vi "Event_Shape_Identifier_2011.vi"() -> ()   [LabVIEW 2011]
uses:
  <vilib>/Analysis/NI_AALPro.lvlib
  <vilib>/Utility/file.llb/Read From Spreadsheet File (string).vi
  <vilib>/Analysis/NI_AAL_SigProc.lvlib
  <vilib>/Analysis/6fits.llb/Curve Fitting Criteria.ctl
panel:
  in  "Header Rows":i32=1
  in  "Events File":path
  out "Event Count":string[][](array[string])
  in  "Tolerance":dbl=3.0
  out "Unique Event Shapes":string[](array[string])
  in  "Sensitivity":dbl=3.0 format="%#_13g"
  out "Peaks Found":i32
  out "Peak Identification":cluster{"Axis":dbl[], dbl[]}[](graph)
  in  "Binsize":i32=20
  out "Output Path (.csv)":path
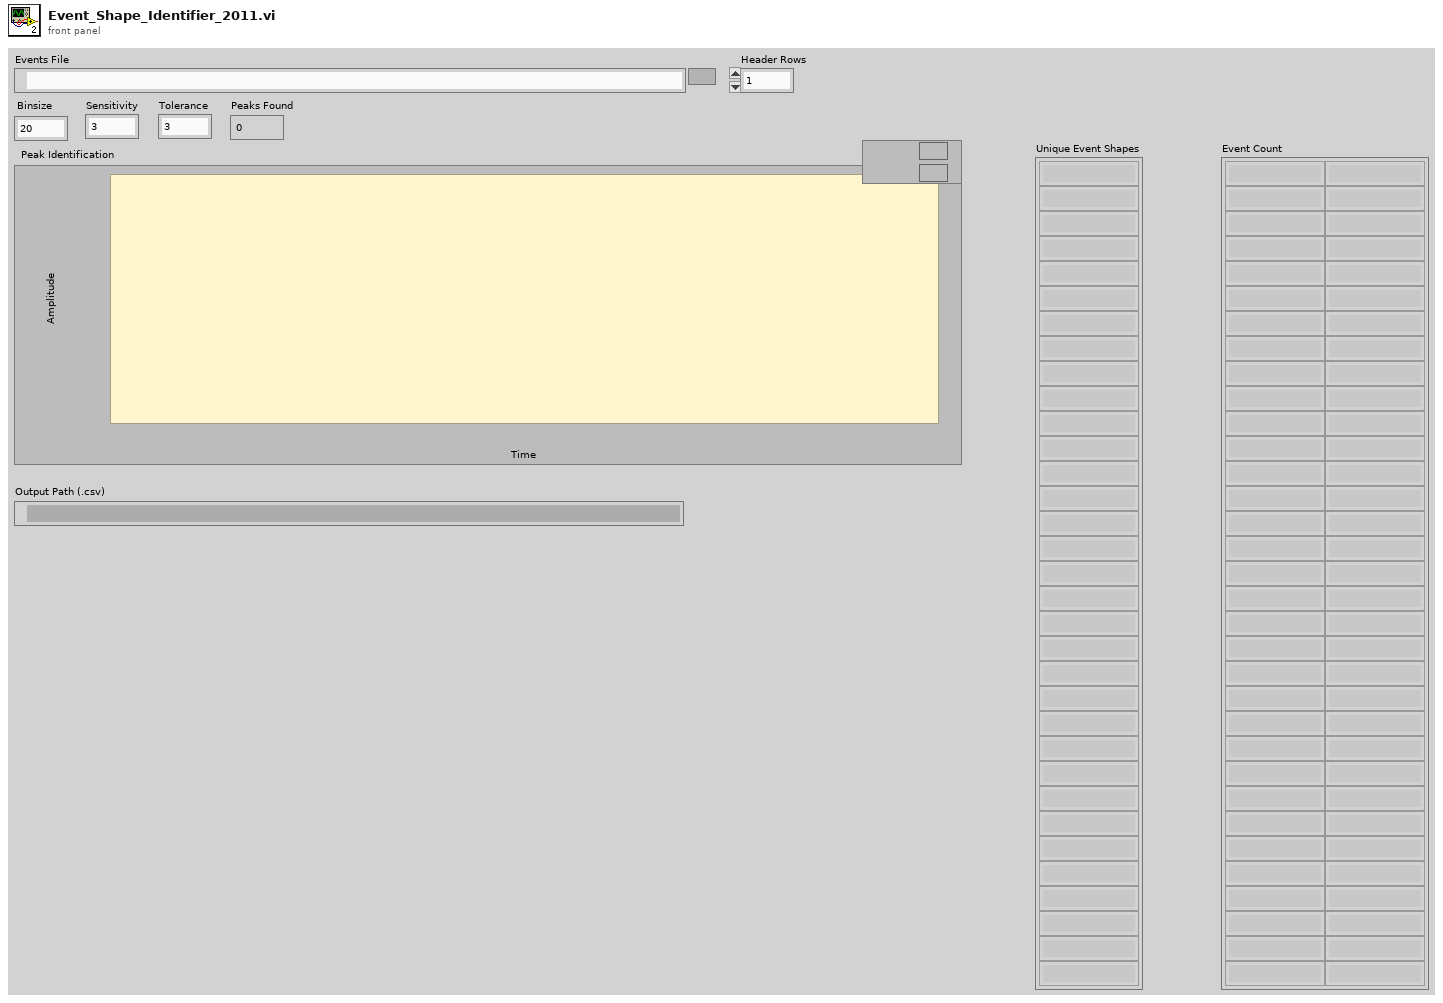
[diagram p1: front panel]
types:
  T1 = typedef "NI_AALPro.lvlib/Curve Fitting Criteria.ctl" = u16
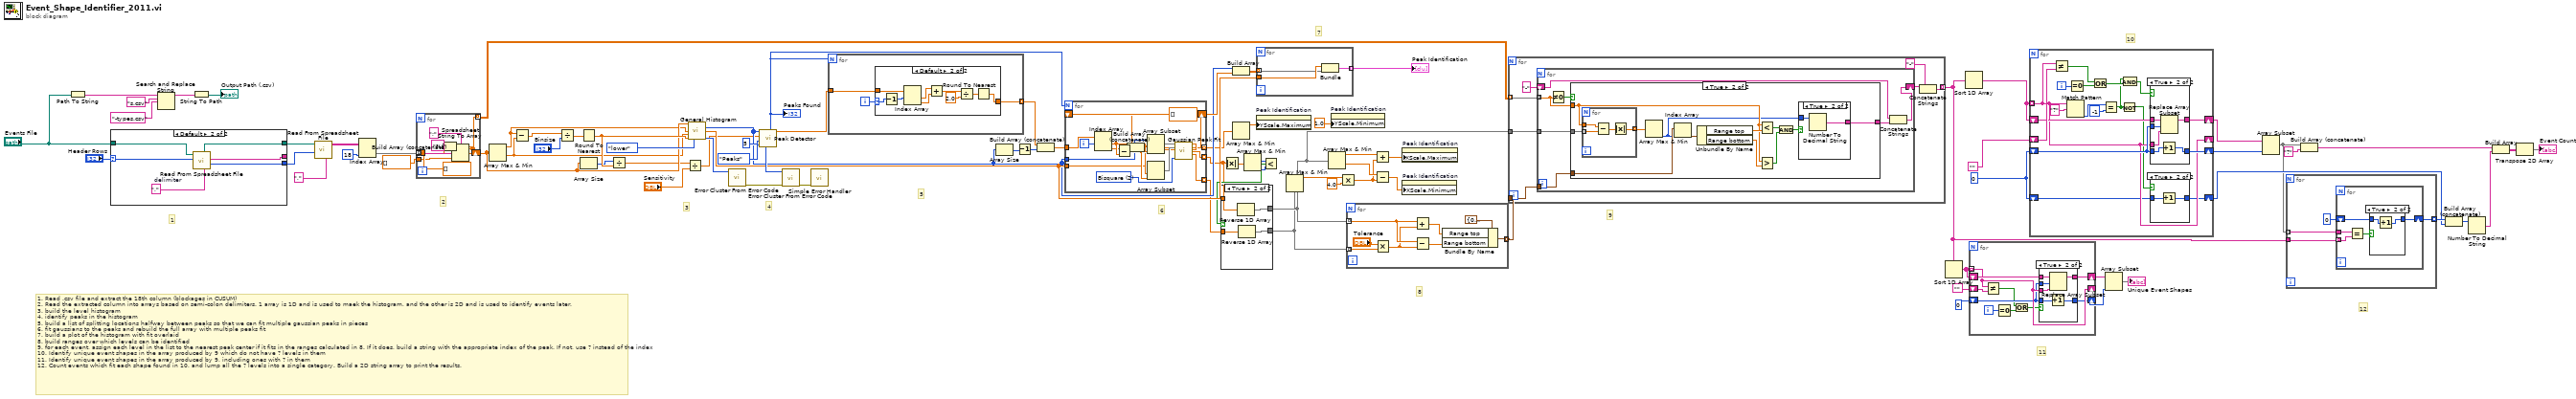
[diagram p0: block diagram]
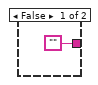
[diagram p7: hidden frame]
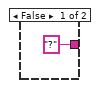
[diagram p8: hidden frame]
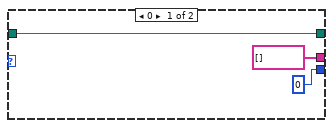
[diagram p10: hidden frame]
diagram:
  w23 = 0
  # "1. Read .csv file and extract the 18th column (blockages in CUSUM)\n2. Read the extracted column into arrays based on semi-colon delimiters. 1 array is 1D and is used to maek the histogram, and the other is 2D and is used to identify events later.\n3. build the level histogram\n4. identify peaks in the histogram\n5. build a list of splitting locations halfway between peaks so that we can fit multiple gaussian peaks in pieces\n6. fit gaussians to the peaks and rebuild the full array with multiple peaks fit\n7. build a plot of the histogram with fit overlaid\n8. build ranges over which levels can be identified\n9. for each event, assign each level in the list to the nearest peak center if it fits in the ranges calculated in 8. If it does, build a string with the appropriate index of the peak. If not, use ? instead of the index\n10. Identify unique event shapes in the array produced by 9 which do not have ? levels in them\n11. Identify unique event shapes in the array produced by 9, including ones with ? in them\n12. Count events which fit each shape found in 10, and lump all the ? levels into a single category. Build a 2D string array to print the results."
  # "12"
  # "11"
  # "10"
  # "9"
  # "8"
  # "7"
  # "6"
  # "5"
  # "4"
  # "3"
  # "2"
  # "1"
  n1 = Path To String(path="Events File") -> (string=w83:string)
  n2 = case shown="Default" "Header Rows" {
    selector: "Header Rows" -> [_ w90]
    tunnel: "Events File" -> [w87 w95]
    tunnel: [string[] [] ("first row") w93] -> _
    tunnel: [0 ("mark after read (chars.)") w92] -> w84
    tunnel: [w87 w91] -> w85
    frame 0 {
    }
    frame Default {
      w94 = ","  # delimiter
      n3 = call-poly <vilib>:"Read From Spreadsheet File.vi"("delimiter (\\t)"=w94, "number of rows (all:-1)"=w90, "file path (dialog if empty)"=w95) -> ("mark after read (chars.)"=w92:i32, "first row"=w93:string[], "new file path (Not A Path if cancelled)"=w91:path)  [unwired: 4 in, 2 out]
    }
  }
  n4 = Search and Replace String(input string=w83, search string="s.csv", replace string="-types.csv" ("replace string (\"\")")) -> (result string=w80:string)  [unwired: 5 in, 3 out]
  n5 = String To Path(string=w80) -> (path=→"Output Path (.csv)":path)
  n6 = call-poly <vilib>:"Read From Spreadsheet File.vi"("delimiter (\\t)"="," ("delimiter (\\t)"), "start of read offset (chars.:0)"=w84, "file path (dialog if empty)"=w85) -> ("all rows"=w65:string[][])  [unwired: 4 in, 4 out]
  n7 = Index Array(array=w65, index (col)=18 ("disabled index (col)")) -> (element=w77:string[])  [unwired: 1 in]
  n8 = for {
    tunnel: w77 -> [w102] mode=indexing
    tunnel: dbl[] [] -> [w99]
    tunnel: [w98] -> w43 mode=indexing
    shift-right: [w96] -> w51
    shift-left: dbl[] [] -> [w97]
    n9 = Spreadsheet String To Array(delimiter (Tab)=";", format string="%f", spreadsheet string=w102, array type (2D Dbl)=w99) -> (array=w98:dbl[])
    n10 = Build Array (concatenate)(w97, w98) -> (w96:dbl[])
  }
  n11 = Array Max & Min(array=w51) -> (max value=w49:dbl, min value=w48:dbl)  [unwired: 2 out]
  n12 = Subtract(x=w49, y=w48) -> (x-y=w52:dbl)
  n13 = Divide(x=w52, y="Binsize") -> (x/y=w47:dbl)
  n14 = Round To Nearest(number=w47) -> (nearest integer value=w76:dbl)
  n15 = Array Size(array=w51) -> (size(s)=w50:i32)
  n16 = Divide(x=w50, y=w76) -> (x/y=w40:dbl)
  n17 = Divide(x=w40, y="Sensitivity") -> (x/y=w38:dbl)
  n18 = call <vilib>:"General Histogram.vi"("X"=w51, "max"=w49, "min"=w48, "# bins"=w76, "inclusion"=enum32{"lower", "upper"}."lower") -> ("Histogram"=w41:i32[], "Axis"=w58:dbl[], "error"=w74:i32)  [unwired: 6 in, 2 out]
  n19 = call <vilib>:"Error Cluster From Error Code.vi"("error code (0)"=w74) -> ("error out"=w11:errorcluster)  [unwired: 8 in]
  n20 = call <vilib>:"Peak Detector.vi"("peaks/valleys"=enum32{"Peaks", "Valleys"}."Peaks", "width"=5, "threshold"=w38, "X"=w41) -> ("error"=w70:i32, "Locations"=w45:dbl[], "# found"=w57:i32)  [unwired: 3 in, 2 out]
  "Peaks Found" <- w57
  n21 = call <vilib>:"Error Cluster From Error Code.vi"("error in (no error)"=w11, "error code (0)"=w70) -> ("error out"=w71:errorcluster)  [unwired: 7 in]
  n22 = call <vilib>:"Simple Error Handler.vi"("error in (no error)"=w71) -> ()  [unwired: 4 in, 5 out]
  n23 = for {
    N: w57 -> [_]
    tunnel: w45 -> [w105]
    tunnel: [w103] -> w56 mode=indexing
    i -> [w104]
    n24 = case shown="Default" w104 {
      selector: w104 -> [w106 w109]
      tunnel: w105 -> [_ w111]
      tunnel: [w106 w107] -> w103
      frame 0 {
      }
      frame Default {
        n25 = Decrement(x=w109) -> (x-1=w108:i32)
        n26 = Index Array(array=w111, index #1=w108) -> (element #1=w115:dbl, element #2=w110:dbl)  [unwired: 1 in]
        n27 = Add(x=w115, y=w110) -> (x+y=w114:dbl)
        n28 = Divide(x=w114, y=2.0) -> (x/y=w112:dbl)
        n29 = Round To Nearest(number=w112) -> (nearest integer value=w107:dbl)
      }
    }
  }
  n30 = Array Size(array=w41) -> (size(s)=w69:i32)
  n31 = Decrement(x=w69) -> (x-1=w68:i32)
  n32 = Build Array (concatenate)(w56, w68) -> (w55:dbl[])
  n33 = for {
    N: w57 -> [_]
    tunnel: w58 -> [w126]
    tunnel: w41 -> [w125]
    tunnel: w55 -> [w124]
    tunnel: [w121] -> w4 mode=indexing
    tunnel: [w120] -> w6 mode=indexing
    tunnel: [w118] -> w36 mode=indexing
    shift-right: [w116] -> w42
    shift-left: dbl[] [] ("Best Gaussian Fit") -> [w117]
    i -> [w128]
    w119 = T1 2 items=["Least Square", "Least Absolute Residual", "Bisquare"] ("method")
    n34 = Index Array(array=w124, index #1=w128) -> (element #1=w127:dbl, element #2=w123:dbl)  [unwired: 1 in]
    n35 = Subtract(x=w123, y=w127) -> (x-y=w130:dbl)
    n36 = Array Subset(array=w125, index=w127, length=w130) -> (w131:i32[])
    n37 = Array Subset(array=w126, index=w127, length=w130) -> (w129:dbl[])
    n38 = call <vilib>:"Gaussian Peak Fit.vi"("Y"=w131, "X"=w129, "method"=w119) -> ("Best Gaussian Fit"=w122:dbl[], "amplitude"=w118:dbl, "center"=w121:dbl, "standard deviation"=w120:dbl)  [unwired: 6 in, 3 out]
    n39 = Build Array (concatenate)(w117, w122) -> (w116:dbl[])
  }
  n40 = Absolute Value(x=w4) -> (abs(x)=w3:dbl[])
  n41 = Build Array(w41, w42) -> (w67:dbl[][])
  n42 = Array Max & Min(array=w36) -> (max value=w35:dbl)  [unwired: 3 out]
  n43 = Array Max & Min(array=w3) -> (max index (indices)=w10:i32, min index (indices)=w9:i32)  [unwired: 2 out]
  n44 = for {
    tunnel: w58 -> [w134]
    tunnel: w67 -> [w133] mode=indexing
    tunnel: [w132] -> w66 mode=indexing
    n45 = Bundle("Axis"=w134, w133) -> (w132:cluster{"Axis":dbl[], dbl[]})  [unwired: 1 in]
  }
  "Peak Identification" <- w66
  n46 = property on="Peak Identification" class="XYGraph (strict)"("YScale.Maximum"=w35) -> ()  [unwired: 2 in, 2 out]
  n47 = Less?(x=w10, y=w9) -> (x < y?=w8:bool)
  n48 = case shown="True" w8 {
    tunnel: w4 -> [w136 w140]
    tunnel: [w136 w139] -> w7
    tunnel: w6 -> [w135 w138]
    tunnel: [w135 w137] -> w5
    frame False {
    }
    frame True {
      n49 = Reverse 1D Array(array=w140) -> (reversed array=w139:dbl[])
      n50 = Reverse 1D Array(array=w138) -> (reversed array=w137:dbl[])
    }
  }
  n51 = Array Max & Min(array=w5) -> (max value=w54:dbl)  [unwired: 3 out]
  n52 = Array Max & Min(array=w7) -> (max value=w63:dbl, min value=w62:dbl)  [unwired: 2 out]
  n53 = property on="Peak Identification" class="XYGraph (strict)"("YScale.Minimum"=1.0 ("Y Scale.Range:Minimum")) -> ()  [unwired: 2 in, 2 out]
  n54 = Multiply(x=w54, y=4.0) -> (x*y=w61:dbl)
  n55 = for {
    tunnel: w7 -> [w147] mode=indexing
    tunnel: w5 -> [w148] mode=indexing
    tunnel: [w143] -> w44 mode=indexing
    n56 = Multiply(x="Tolerance", y=w148) -> (x*y=w146:dbl)
    n57 = Add(x=w147, y=w146) -> (x+y=w141:dbl)
    n58 = Subtract(x=w147, y=w146) -> (x-y=w144:dbl)
    n59 = Bundle By Name(cluster=cluster{"Range top":dbl, "Range bottom":dbl} {"Range top"=0.0, "Range bottom"=0.0} ("Cluster"), "Range top"=w141, "Range bottom"=w144) -> (w143:cluster{"Range top":dbl, "Range bottom":dbl})
  }
  n60 = Add(x=w63, y=w61) -> (x+y=w60:dbl)
  n61 = Subtract(x=w62, y=w61) -> (x-y=w59:dbl)
  n62 = property on="Peak Identification" class="XYGraph (strict)"("XScale.Maximum"=w60) -> ()  [unwired: 2 in, 2 out]
  n63 = property on="Peak Identification" class="XYGraph (strict)"("XScale.Minimum"=w59) -> ()  [unwired: 2 in, 2 out]
  n64 = for {
    tunnel: w43 -> [w155] mode=indexing
    tunnel: w44 -> [w154]
    tunnel: w7 -> [w153]
    tunnel: [w149] -> w24 mode=indexing
    n65 = for {
      tunnel: w155 -> [w160] mode=indexing
      tunnel: w154 -> [w161]
      tunnel: w153 -> [w162]
      shift-right: [w158] -> w151
      shift-left: "-" -> [w157]
      n66 = Not Equal To 0?(x=w160) -> (x != 0?=w159:bool)
      n67 = case shown="True" w159 {
        tunnel: w162 -> [_ w175]
        tunnel: w161 -> [_ w173]
        tunnel: w160 -> [_ w170]
        tunnel: ["" w164] -> w156
        frame False {
        }
        frame True {
          n68 = for {
            tunnel: w170 -> [w182]
            tunnel: w175 -> [w181] mode=indexing
            tunnel: [w179] -> w174 mode=indexing
            n69 = Subtract(x=w182, y=w181) -> (x-y=w180:dbl)
            n70 = Absolute Value(x=w180) -> (abs(x)=w179:dbl)
          }
          n71 = Array Max & Min(array=w174) -> (min index (indices)=w165:i32)  [unwired: 3 out]
          n72 = Index Array(array=w173, index=w165) -> (element=w172:cluster{"Range top":dbl, "Range bottom":dbl})
          n73 = Unbundle By Name(w172) -> ("Range top"=w171:dbl, "Range bottom"=w169:dbl)
          n74 = Less?(x=w170, y=w171) -> (x < y?=w168:bool)
          n75 = Greater?(x=w170, y=w169) -> (0:w167:bool)
          n76 = And(x=w168, y=w167) -> (x .and. y?=w166:bool)
          n77 = case shown="True" w166 {
            tunnel: w165 -> [_ w178]
            tunnel: ["?" w177] -> w164
            frame False {
            }
            frame True {
              n78 = Number To Decimal String(number=w178) -> (decimal integer string=w177:string)  [unwired: 1 in]
            }
          }
        }
      }
      n79 = Concatenate Strings(w157, w156) -> (w158:string)
    }
    n80 = Concatenate Strings(w151, "-" ("string")) -> (w149:string)
  }
  n81 = Sort 1D Array(array=w24) -> (sorted array=w33:string[])
  n82 = Sort 1D Array(array=w24) -> (sorted array=w29:string[])
  n83 = for {
    shift-right: [w187] -> w32
    shift-left: w33 -> [w191]
    shift-right: [w188] -> w31
    shift-left: 0 -> [w189]
    tunnel: w33 -> [w190] mode=indexing
    shift-right: [w190] -> _
    shift-left: "" -> [w192]
    i -> [w186]
    n84 = Not Equal?(x=w190, y=w192) -> (x != y?=w185:bool)
    n85 = Equal To 0?(x=w186) -> (x = 0?=w184:bool)
    n86 = Or(x=w185, y=w184) -> (x .or. y?=w183:bool)
    n87 = case shown="True" w183 {
      tunnel: w191 -> [w194 w200]
      tunnel: w189 -> [_ w199]
      tunnel: w190 -> [_ w198]
      tunnel: w189 -> [w193 w197]
      tunnel: [w193 w196] -> w188
      tunnel: [w194 w195] -> w187
      frame False {
      }
      frame True {
        n88 = Increment(x=w197) -> (x+1=w196:i32)
        n89 = Replace Array Subset(array=w200, new element=w198, index=w199) -> (w195:string[])
      }
    }
  }
  n90 = for {
    shift-right: [w214] -> w28
    shift-left: w29 -> [w217]
    shift-right: [w215] -> w27
    shift-left: w23 -> [w216]
    tunnel: w29 -> [w210] mode=indexing
    shift-right: [w210] -> _
    shift-left: "" -> [w218]
    shift-right: [w201] -> w21
    shift-left: w23 -> [w202]
    i -> [w213]
    n91 = Not Equal?(x=w210, y=w218) -> (x != y?=w212:bool)
    n92 = Match Pattern(string=w210, regular expression="?") -> (offset past match=w208:i32)  [unwired: 1 in, 3 out]
    n93 = Equal To 0?(x=w213) -> (x = 0?=w211:bool)
    n94 = Or(x=w212, y=w211) -> (x .or. y?=w206:bool)
    n95 = Equal?(x=w208, y=-1) -> (x = y?=w204:bool)
    n96 = Not(x=w204) -> (.not. x?=w203:bool)
    n97 = And(x=w204, y=w206) -> (x .and. y?=w205:bool)
    n98 = case shown="True" w205 {
      tunnel: w217 -> [w223 w229]
      tunnel: w216 -> [_ w228]
      tunnel: w210 -> [_ w227]
      tunnel: w216 -> [w222 w226]
      tunnel: [w222 w225] -> w215
      tunnel: [w223 w224] -> w214
      frame False {
      }
      frame True {
        n99 = Increment(x=w226) -> (x+1=w225:i32)
        n100 = Replace Array Subset(array=w229, new element=w227, index=w228) -> (w224:string[])
      }
    }
    n101 = case shown="True" w203 {
      tunnel: w202 -> [w219 w221]
      tunnel: [w219 w220] -> w201
      frame False {
      }
      frame True {
        n102 = Increment(x=w221) -> (x+1=w220:i32)
      }
    }
  }
  n103 = Array Subset(array=w32, length=w31) -> (→"Unique Event Shapes":string[])  [unwired: 1 in]
  n104 = Array Subset(array=w28, length=w27) -> (w20:string[])  [unwired: 1 in]
  n105 = for {
    tunnel: w20 -> [w233] mode=indexing
    tunnel: w24 -> [w232]
    tunnel: [w230] -> w22 mode=indexing
    n106 = for {
      tunnel: w233 -> [w235]
      tunnel: w232 -> [w234] mode=indexing
      shift-right: [w236] -> w230
      shift-left: 0 ("x") -> [w237]
      n107 = Equal?(x=w235, y=w234) -> (x = y?=w238:bool)
      n108 = case shown="True" w238 {
        tunnel: w237 -> [w239 w241]
        tunnel: [w239 w240] -> w236
        frame False {
        }
        frame True {
          n109 = Increment(x=w241) -> (x+1=w240:i32)
        }
      }
    }
  }
  n110 = Build Array (concatenate)(w20, "?" ("regular expression")) -> (w17:string[])
  n111 = Build Array (concatenate)(w22, w21) -> (w18:i32[])
  n112 = Number To Decimal String(number=w18) -> (decimal integer string=w16:string[])  [unwired: 1 in]
  n113 = Build Array(w17, w16) -> (w15:string[][])
  n114 = Transpose 2D Array(2D array=w15) -> (transposed array=→"Event Count":string[][])
